vi "Calculate Transform.vi"(11 "all rows":dbl[][](array[numeric])) -> ()   [LabVIEW 2015]
uses:
  Globals.vi
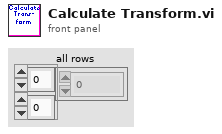
[diagram p1: front panel]
types:
  T1 = cluster{"x shift":dbl, "y shift":dbl, "z shift":dbl, "Theta x":dbl, "Theta y":dbl}
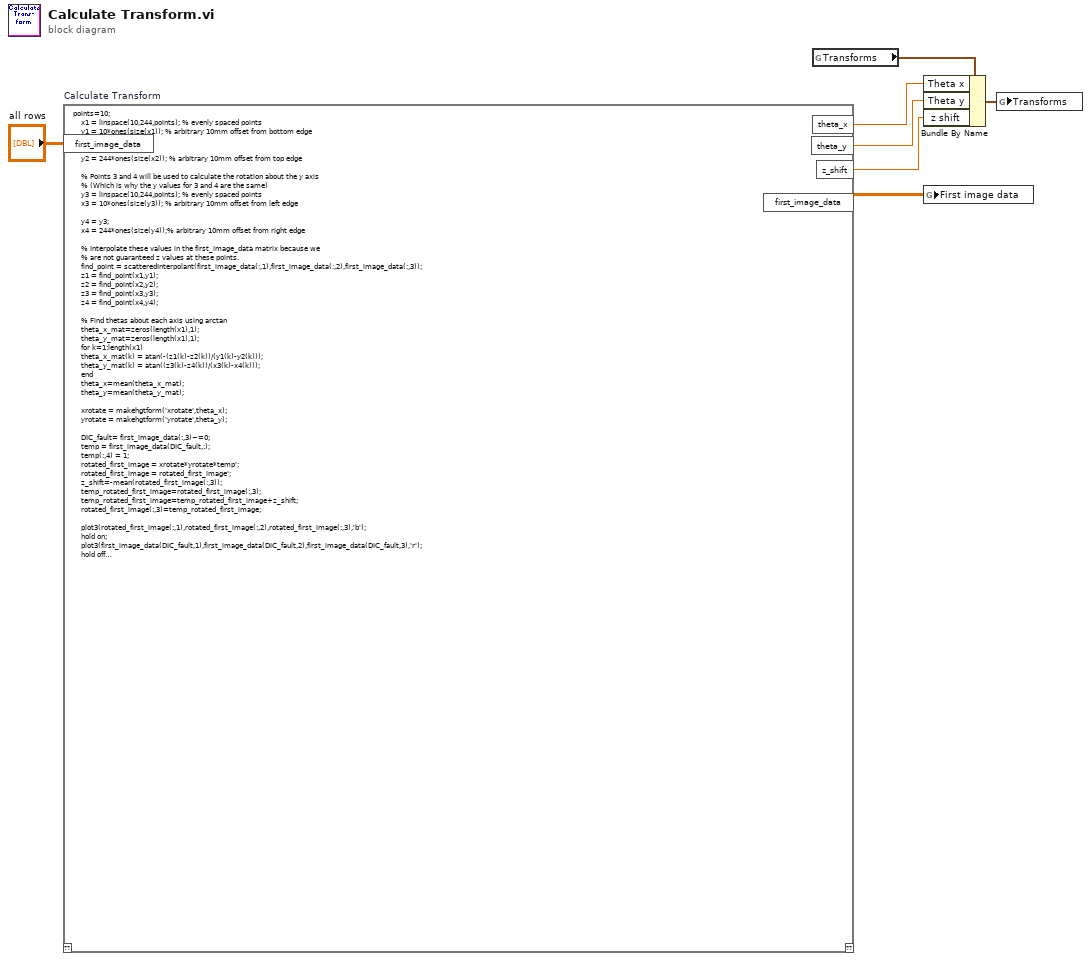
[diagram p0: block diagram]
diagram:
  n1 = script code="points=10;\n    x1 = linspace(10,244,points); % evenly spaced points\n    y1 = 10*ones(size(x1)); % arbitrary 10mm offset from bottom edge\n    \n    x2 = x1;\n    y2 = 244*ones(size(x2)); % arbitrary 10mm offset from top edge\n    \n    % Points 3 and 4 will be used to calculate the rotation about the y axis\n    % (Which is why the y values for 3 and 4 are the same)\n    y3 = linspace(10,244,points); % evenly spaced points \n    x3 = 10*ones(size(y3)); % arbitrary 10mm offset from left edge\n    \n    y4 = y3;\n    x4 = 244*ones(size(y4));% arbitrary 10mm offset from right edge\n        \n    % Interpolate these values in the first_image_data matrix because we\n    % are not guaranteed z values at these points.\n    find_point = scatteredInterpolant(first_image_data(:,1),first_image_data(:,2),first_image_data(:,3));\n    z1 = find_point(x1,y1);\n    z2 = find_point(x2,y2);\n    z3 = find_point(x3,y3);\n    z4 = find_point(x4,y4);\n\n    % Find thetas about each axis using arctan\n    theta_x_mat=zeros(length(x1),1);\n    theta_y_mat=zeros(length(x1),1);\n    for k=1:length(x1)\n    theta_x_mat(k) = atan(-(z1(k)-z2(k))/(y1(k)-y2(k)));    \n    theta_y_mat(k) = atan((z3(k)-z4(k))/(x3(k)-x4(k)));\n    end\n    theta_x=mean(theta_x_mat);\n    theta_y=mean(theta_y_mat);\n    \n    xrotate = makehgtform('xrotate',theta_x);\n    yrotate = makehgtform('yrotate',theta_y);\n    \n    DIC_fault= first_image_data(:,3)~=0;\n    temp = first_image_data(DIC_fault,:);\n    temp(:,4) = 1;\n    rotated_first_image = xrotate*yrotate*temp';\n    rotated_first_image = rotated_first_image';\n    z_shift=-mean(rotated_first_image(:,3));\n    temp_rotated_first_image=rotated_first_image(:,3);\n    temp_rotated_first_image=temp_rotated_first_image+z_shift;\n    rotated_first_image(:,3)=temp_rotated_first_image;\n \n    plot3(rotated_first_image(:,1),rotated_first_image(:,2),rotated_first_image(:,3),'b');\n    hold on;\n    plot3(first_image_data(DIC_fault,1),first_image_data(DIC_fault,2),first_image_data(DIC_fault,3),'r');\n    hold off;\n    xlabel('X (mm)');\n    ylabel('Y (mm)');\n    zlabel('Z (mm)');" "Calculate Transform"("first_image_data"="all rows") -> ("theta_y"=w5:dbl, "theta_x"=w4:dbl, "z_shift"=w6:dbl, "first_image_data"=w7:dbl[][])  [unwired: 1 in, 1 out]
  n2 = global read "Globals.vi" "Transforms"() -> (w3:T1)
  n3 = Bundle By Name(cluster=w3, "Theta x"=w4, "Theta y"=w5, "z shift"=w6) -> (w2:T1)
  n4 = global write "Globals.vi" "First image data"(w7) -> ()
  n5 = global write "Globals.vi" "Transforms"(w2) -> ()
